vi "gfitsio-open-create-replace-image.vi"(4 "image data type":T1 items=["<invalid type>"=0, "BYTE_IMG  (U8)"=8, "SHORT_IMG  (I16)"=16, "USHORT_IMG  (U16)"=20, "LONG_IMG  (I32)"=32, "ULONG_IMG  (U32)"=40, "FLOAT_IMG  (SGL)"=-32, "DOUBLE_IMG  (DBL)"=-64], 5 "prompt (\"Select an HDU\")":string="Select an HDU", 6 "advisory dialog? (display:T)":bool=TRUE, 7 "hdu name (dialog if empty)":string, 8 "error in (no error)":errorcluster, 9 "function (open or create)":T3(ring)=enum."open or create", 10 "naxes":i32[](array[numeric]), 11 "gfits refnum":T2) -> (0 "error out":errorcluster, 2 "hdu name out":string, 3 "dup gfits refnum":T2)   [LabVIEW 2019, in "gfitsio.lvlib"]
doc: "Opens an existing FITS image HDU, creates a new FITS image HDU, or replaces an existing FITS image HDU, programmatically or interactively using a dialog box. You can optionally specify a dialog prompt."
uses:
  gfitsio.lvlib
  gfitsio-refnum.ctl
  cfitsio-bitpix.ctl
  cfitsio-hdutypes.ctl
  gfitsio-error-codes.ctl
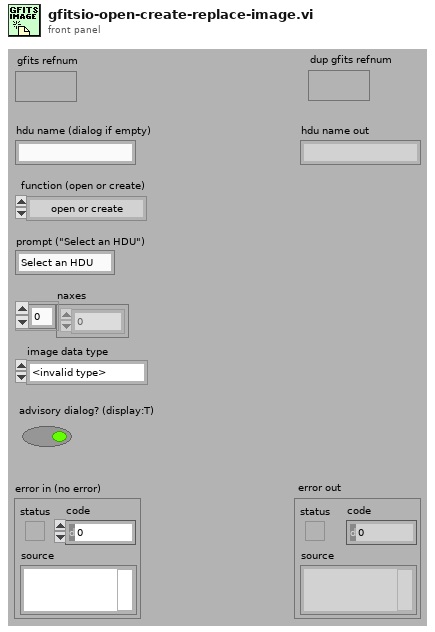
[diagram p1: front panel]
types:
  T1 = typedef "gfitsio.lvlib/cfitsio-bitpix.ctl" = i32
  T2 = typedef "gfitsio.lvlib/gfitsio-refnum.ctl" = refnum<k1>
  T3 = enum16{"open", "open or create", "create", "create or replace"}
  T4 = typedef "gfitsio.lvlib/cfitsio-hdutypes.ctl" = i32
  T5 = typedef "gfitsio.lvlib/gfitsio-error-codes.ctl" = i32
  T6 = enum16{"Error", "Ok", "Cancel", "Abort", "Retry", "Ignore", "Yes", "No", "Close", "Help", "Disabled"}
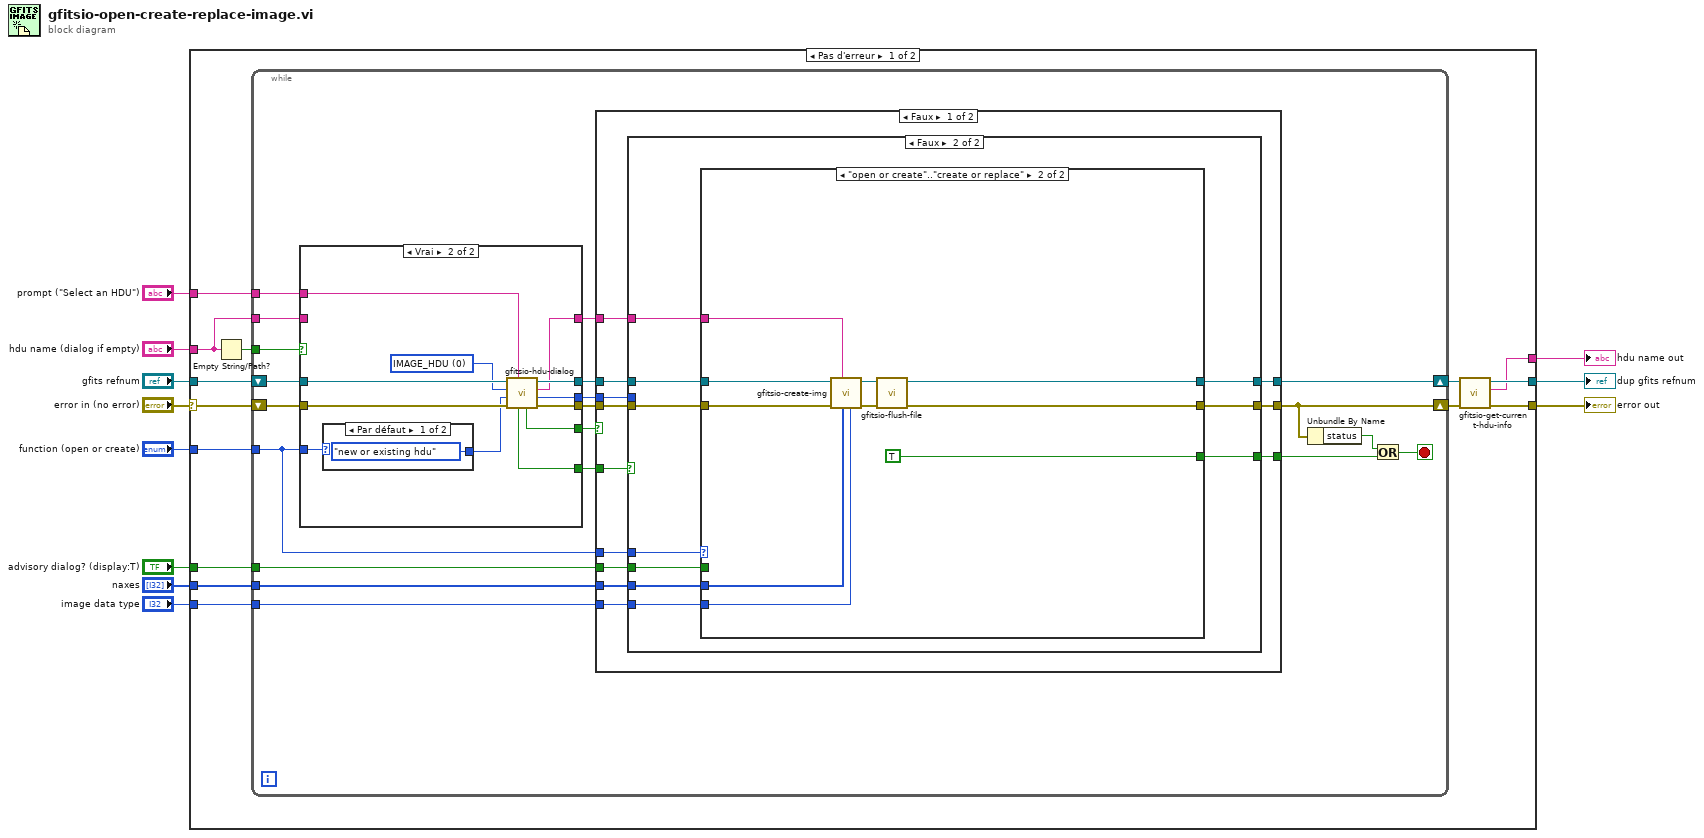
[diagram p0: block diagram]
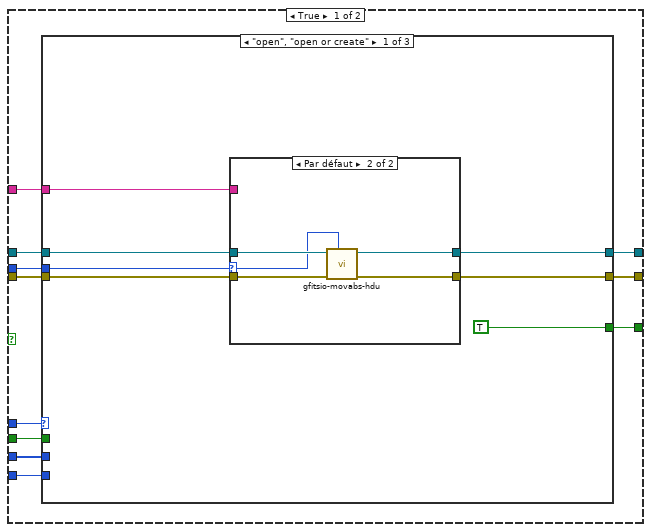
[diagram p2: hidden frame]
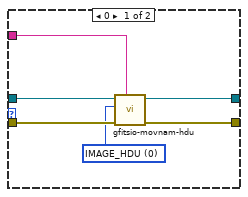
[diagram p3: hidden frame]
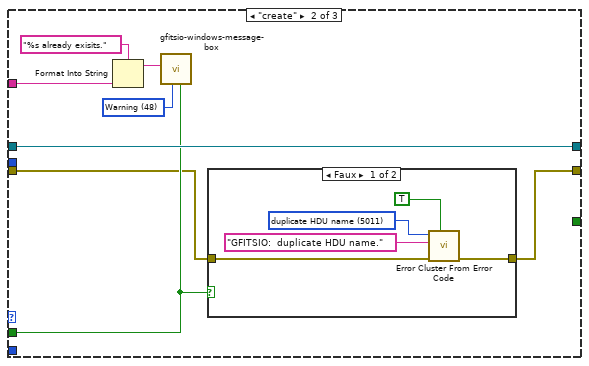
[diagram p4: hidden frame]
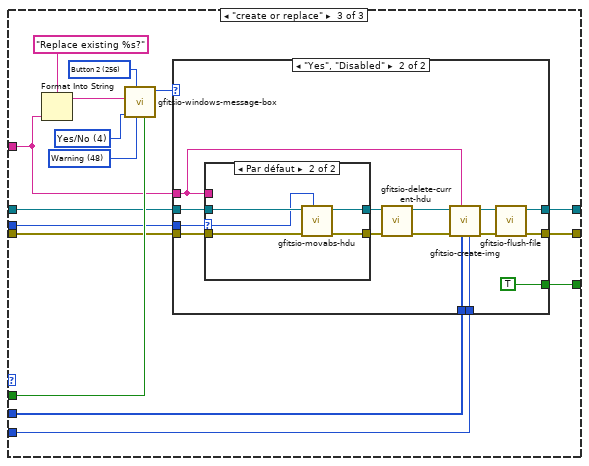
[diagram p6: hidden frame]
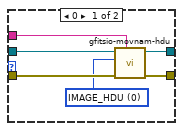
[diagram p8: hidden frame]
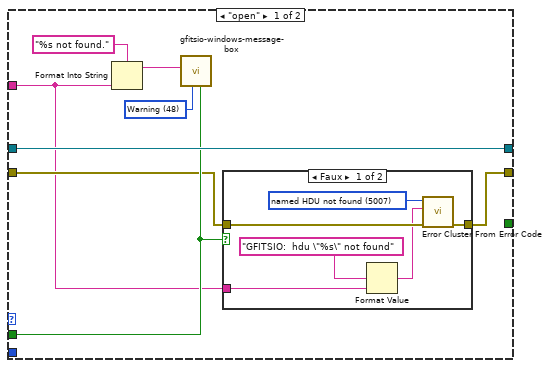
[diagram p9: hidden frame]
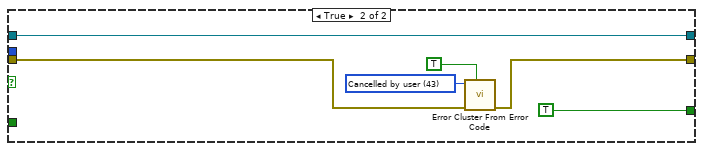
[diagram p11: hidden frame]
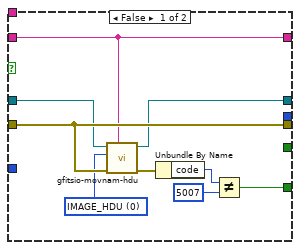
[diagram p12: hidden frame]
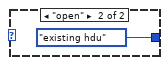
[diagram p13: hidden frame]
diagram:
  n1 = case shown="Pas d'erreur" "error in (no error)" {
    selector: "error in (no error)" -> [w12 w209]
    tunnel: "advisory dialog? (display:T)" -> [w24 _]
    tunnel: "function (open or create)" -> [w23 _]
    tunnel: "prompt (\"Select an HDU\")" -> [w22 _]
    tunnel: "hdu name (dialog if empty)" -> [w21 _]
    tunnel: "gfits refnum" -> [w20 w210]
    tunnel: [w17 w209] -> w6
    tunnel: [w16 w210] -> w5
    tunnel: [w15 _] -> w4
    tunnel: "naxes" -> [w14 _]
    tunnel: "image data type" -> [w13 _]
    frame No Error {
      n2 = Empty String/Path?(string/path=w21) -> (empty?=w25:bool)
      n3 = while {
        tunnel: w23 -> [w29]
        tunnel: w25 -> [w43]
        shift-right: [w38] -> w18
        shift-left: w12 -> [w45]
        shift-right: [w41] -> w19
        shift-left: w20 -> [w44]
        tunnel: w21 -> [w33]
        tunnel: w22 -> [w30]
        tunnel: w24 -> [w28]
        tunnel: w14 -> [w27]
        tunnel: w13 -> [w26]
        stop <- w35 stop-if-true
        n4 = case shown="Vrai" w43 {
          tunnel: [w194 w206] -> w40
          tunnel: [w192 w205] -> w42
          tunnel: w45 -> [w194 w204]
          tunnel: w44 -> [w193 w203]
          tunnel: w29 -> [_ w202]
          tunnel: [_ w201] -> w39
          tunnel: [w188 w200] -> w34
          tunnel: w33 -> [w187 _]
          tunnel: [w187 w199] -> w32
          tunnel: [_ w198] -> w31
          tunnel: w30 -> [_ w197]
          frame False {
            w186 = T4 0 items=["ANY_HDU"=-1, "IMAGE_HDU"=0, "ASCII_TBL"=1, "BINARY_TBL"=2] ("hdu type (ANY)")
            n5 = call "gfitsio-movnam-hdu.vi"("extname"=w187, "error in (no error)"=w194, "hdutype (ANY_HDU)"=w186, "gfits refnum"=w193) -> ("error out"=w191:errorcluster, "dup gfits refnum"=w192:T2)  [unwired: 6 in]
            n6 = Unbundle By Name(w191) -> ("code"=w190:i32)
            n7 = Not Equal?(x=w190, y=5007) -> (x != y?=w188:bool)
          }
          frame True {
            w195 = T4 0 items=["ANY_HDU"=-1, "IMAGE_HDU"=0, "ASCII_TBL"=1, "BINARY_TBL"=2] ("hdu type (ANY)")
            n8 = case shown="Par défaut" w202 {
              tunnel: [enum32{"existing hdu", "new or existing hdu"}."new or existing hdu" ("select mode (new or existing)") enum32{"existing hdu", "new or existing hdu"}."existing hdu" ("select mode (new or existing)")] -> w196
              frame Default {
              }
              frame "open" {
              }
            }
            n9 = call "gfitsio-hdu-dialog.vi"("prompt (\"Select an HDU\")"=w197, "error in (no error)"=w204, "select mode (new or existing)"=w196, "hdu type (ANY_HDU)"=w195, "gfits refnum"=w203) -> ("error out"=w206:errorcluster, "hdu number (0 if cancelled)"=w198:i32, "hdu name (\"\" if cancelled)"=w199:string, "dup gfits refnum"=w205:T2, "cancelled"=w201:bool, "exists"=w200:bool)  [unwired: 1 in]
          }
        }
        n10 = case shown="Faux" w39 {
          tunnel: w42 -> [w57 w185]
          tunnel: [w54 w185] -> w41
          tunnel: w40 -> [w56 w181]
          tunnel: [w55 w180] -> w38
          tunnel: [w48 TRUE] -> w36
          tunnel: w34 -> [w53 _]
          tunnel: w32 -> [w51 _]
          tunnel: w31 -> [w50 _]
          tunnel: w29 -> [w52 _]
          tunnel: w28 -> [w49 _]
          tunnel: w27 -> [w47 _]
          tunnel: w26 -> [w46 _]
          frame False {
            n11 = case shown="Faux" w53 {
              tunnel: w57 -> [w67 w153]
              tunnel: w56 -> [w64 w152]
              tunnel: [w65 w151] -> w55
              tunnel: [w66 w150] -> w54
              tunnel: w52 -> [w68 w154]
              tunnel: w51 -> [w63 w148]
              tunnel: w50 -> [w62 _]
              tunnel: w49 -> [w61 w149]
              tunnel: [w60 w147] -> w48
              tunnel: w47 -> [w59 w146]
              tunnel: w46 -> [w58 w145]
              frame True {
                n12 = case shown="\"open\", \"open or create\"" w68 {
                  tunnel: w67 -> [w74 w94 w110]
                  tunnel: [w72 w94 w109] -> w66
                  tunnel: [w73 w87 w107] -> w65
                  tunnel: w64 -> [w75 w88 w108]
                  tunnel: w63 -> [w71 w90 w104]
                  tunnel: w62 -> [w70 _ w103]
                  tunnel: w61 -> [_ w89 w111]
                  tunnel: [TRUE _ w105] -> w60
                  tunnel: w59 -> [_ _ w102]
                  tunnel: w58 -> [_ _ w101]
                  frame "open", "open or create" {
                    n13 = case shown="Par défaut" w70 {
                      selector: w70 -> [_ w82]
                      tunnel: w75 -> [w81 w85]
                      tunnel: w74 -> [w80 w86]
                      tunnel: [w79 w84] -> w73
                      tunnel: [w78 w83] -> w72
                      tunnel: w71 -> [w77 _]
                      frame 0 {
                        w76 = T4 0 items=["ANY_HDU"=-1, "IMAGE_HDU"=0, "ASCII_TBL"=1, "BINARY_TBL"=2] ("hdu type (ANY)")
                        n14 = call "gfitsio-movnam-hdu.vi"("extname"=w77, "error in (no error)"=w81, "hdutype (ANY_HDU)"=w76, "gfits refnum"=w80) -> ("error out"=w79:errorcluster, "dup gfits refnum"=w78:T2)  [unwired: 6 in]
                      }
                      frame Default {
                        n15 = call "gfitsio-movabs-hdu.vi"("hdunum"=w82, "error in (no error)"=w85, "gfits refnum"=w86) -> ("error out"=w84:errorcluster, "dup gfits refnum"=w83:T2)  [unwired: 6 in, 1 out]
                      }
                    }
                  }
                  frame "create" {
                    w91 = u32 48 items=["None"=0, "Warning"=48, "Confirmation"=64, "Question"=32, "Error"=16, "User Icon"=128] ("Icon (None)")
                    n16 = Format Into String(format string="%s already exisits.", w90) -> (resulting string=w92:string)  [unwired: 2 in, 1 out]
                    n17 = call "gfitsio-windows-message-box.vi"("enable dialog?"=w89, "Icon (None)"=w91, "Text"=w92) -> ()  [unwired: 8 in, 1 out]
                    n18 = case shown="Faux" w89 {
                      tunnel: w88 -> [w99 w100]
                      tunnel: [w98 w100] -> w87
                      frame False {
                        w95 = T5 5011 items=["no error"=0, "dimensionality conflict"=5001, "fpixel out of image bounds"=5002, "lpixel out of image bounds"=5003, "increment size larger than image"=5004, "increment must be greater than zero"=5005, "fpixel must specify lower left corner"=5006, "named HDU not found"=5007, "specified row is past the end of the table"=5008, "wrong number of elements for column"=5009, "column is not scalar"=5010, "duplicate HDU name"=5011, "invalid table type"=5012] ("Ring")
                        n19 = call <vilib>:"Error Cluster From Error Code.vi"("show call chain? (False)"=TRUE, "error in (no error)"=w99, "error message (\"\")"="GFITSIO:  duplicate HDU name." ("error message (\"\")"), "error code (0)"=w95) -> ("error out"=w98:errorcluster)  [unwired: 5 in]
                      }
                      frame True {
                      }
                    }
                  }
                  frame "create or replace" {
                    w113 = u32 256 items=["Button 1"=0, "Button 2"=256, "Button 3"=512, "Button 4"=1024] ("Default (Button 1)")
                    w114 = u32 4 items=["Abort/Retry/Ignore"=2, "OK"=0, "OK/Cancel"=1, "Retry/Cancel"=5, "Yes/No"=4, "Yes/No/Cancel"=3] ("Buttons (OK)")
                    w115 = u32 48 items=["None"=0, "Warning"=48, "Confirmation"=64, "Question"=32, "Error"=16, "User Icon"=128] ("Icon (None)")
                    n20 = Format Into String(format string="Replace existing %s?", w104) -> (resulting string=w112:string)  [unwired: 2 in, 1 out]
                    n21 = call "gfitsio-windows-message-box.vi"("enable dialog?"=w111, "Icon (None)"=w115, "Default (Button 1)"=w113, "Buttons (OK)"=w114, "Text"=w112) -> ("Button Selected"=w106:T6)  [unwired: 6 in]
                    n22 = case shown="\"Yes\", \"Disabled\"" w106 {
                      tunnel: w110 -> [w118 w132]
                      tunnel: [w118 w123] -> w109
                      tunnel: w108 -> [w117 w131]
                      tunnel: [w117 w122] -> w107
                      tunnel: [_ TRUE] -> w105
                      tunnel: w104 -> [_ w121]
                      tunnel: w103 -> [_ w130]
                      tunnel: w102 -> [_ w120]
                      tunnel: w101 -> [_ w119]
                      frame "No", Default {
                      }
                      frame "Yes", "Disabled" {
                        n23 = case shown="Par défaut" w130 {
                          selector: w130 -> [_ w140]
                          tunnel: w131 -> [w139 w143]
                          tunnel: w132 -> [w138 w144]
                          tunnel: [w137 w142] -> w129
                          tunnel: [w136 w141] -> w128
                          tunnel: w121 -> [w135 _]
                          frame 0 {
                            w134 = T4 0 items=["ANY_HDU"=-1, "IMAGE_HDU"=0, "ASCII_TBL"=1, "BINARY_TBL"=2] ("hdu type (ANY)")
                            n24 = call "gfitsio-movnam-hdu.vi"("extname"=w135, "error in (no error)"=w139, "hdutype (ANY_HDU)"=w134, "gfits refnum"=w138) -> ("error out"=w137:errorcluster, "dup gfits refnum"=w136:T2)  [unwired: 6 in]
                          }
                          frame Default {
                            n25 = call "gfitsio-movabs-hdu.vi"("hdunum"=w140, "error in (no error)"=w143, "gfits refnum"=w144) -> ("error out"=w142:errorcluster, "dup gfits refnum"=w141:T2)  [unwired: 6 in, 1 out]
                          }
                        }
                        n26 = call "gfitsio-delete-current-hdu.vi"("error in (no error)"=w129, "gfits refnum"=w128) -> ("error out"=w126:errorcluster, "dup gfits refnum"=w127:T2)  [unwired: 8 in]
                        n27 = call "gfitsio-create-img.vi"("image data type"=w119, "naxes"=w120, "extname"=w121, "error in (no error)"=w126, "gfits refnum"=w127) -> ("error out"=w125:errorcluster, "dup gfits refnum"=w124:T2)  [unwired: 5 in]
                        n28 = call "gfitsio-flush-file.vi"("error in (no error)"=w125, "gfits refnum"=w124) -> ("error out"=w122:errorcluster, "dup gfits refnum"=w123:T2)  [unwired: 8 in]
                      }
                    }
                  }
                }
              }
              frame False {
                n29 = case shown="\"open or create\"..\"create or replace\"" w154 {
                  tunnel: w153 -> [w162 w178]
                  tunnel: w152 -> [w157 w179]
                  tunnel: [w156 w174] -> w151
                  tunnel: [w162 w173] -> w150
                  tunnel: w149 -> [w158 _]
                  tunnel: w148 -> [w155 w172]
                  tunnel: [_ TRUE] -> w147
                  tunnel: w146 -> [_ w171]
                  tunnel: w145 -> [_ w170]
                  frame "open" {
                    w159 = u32 48 items=["None"=0, "Warning"=48, "Confirmation"=64, "Question"=32, "Error"=16, "User Icon"=128] ("Icon (None)")
                    n30 = Format Into String(format string="%s not found.", w155) -> (resulting string=w160:string)  [unwired: 2 in, 1 out]
                    n31 = call "gfitsio-windows-message-box.vi"("enable dialog?"=w158, "Icon (None)"=w159, "Text"=w160) -> ()  [unwired: 8 in, 1 out]
                    n32 = case shown="Faux" w158 {
                      tunnel: w157 -> [w168 w169]
                      tunnel: [w167 w169] -> w156
                      tunnel: w155 -> [w165 _]
                      frame False {
                        w163 = T5 5007 items=["no error"=0, "dimensionality conflict"=5001, "fpixel out of image bounds"=5002, "lpixel out of image bounds"=5003, "increment size larger than image"=5004, "increment must be greater than zero"=5005, "fpixel must specify lower left corner"=5006, "named HDU not found"=5007, "specified row is past the end of the table"=5008, "wrong number of elements for column"=5009, "column is not scalar"=5010, "duplicate HDU name"=5011, "invalid table type"=5012] ("Ring")
                        n33 = Format Value(format string="GFITSIO:  hdu \"%s\" not found", value (0)=w165) -> (output string=w164:string)  [unwired: 1 in]
                        n34 = call <vilib>:"Error Cluster From Error Code.vi"("error in (no error)"=w168, "error message (\"\")"=w164, "error code (0)"=w163) -> ("error out"=w167:errorcluster)  [unwired: 6 in]
                      }
                      frame True {
                      }
                    }
                  }
                  frame "open or create".."create or replace" {
                    n35 = call "gfitsio-create-img.vi"("image data type"=w170, "naxes"=w171, "extname"=w172, "error in (no error)"=w179, "gfits refnum"=w178) -> ("error out"=w176:errorcluster, "dup gfits refnum"=w175:T2)  [unwired: 5 in]
                    n36 = call "gfitsio-flush-file.vi"("error in (no error)"=w176, "gfits refnum"=w175) -> ("error out"=w174:errorcluster, "dup gfits refnum"=w173:T2)  [unwired: 8 in]
                  }
                }
              }
            }
          }
          frame True {
            w183 = 43 items=["No error", "Argument error", "Memory is full", "Out of zone", "End of file", "File already open", "Generic file I/O error", "File not found", "File permission error", "Disk is full", "Duplicate path", "Too many files open", "System feature not enabled", "Resource file not found", "Cannot add resource", "Resource not found", "Image not found", "Image memory error", "Pen does not exist", "Config type invalid", "Config token not found", "Config parse error", "Config memory error", "Bad external code format", "Bad external code offset", "External code not present", "Null window", "Destroy window error", "Null menu", "Print aborted", "Bad print record", "Print driver error", "Windows error during printing", "Memory error during printing", "Print dialog error", "Generic print error", "Invalid device refnum", "Device not found", "Device parameter error", "Device unit error", "Cannot open device", "Device call aborted", "Generic error", "Cancelled by user", "Object ID too low", "Object ID too high", "Object not in heap", "Unknown heap", "Unknown object (invalid DefProc)", "Unknown object (DefProc not in table)", "Message out of range", "Invalid (null) method", "Unknown message", "Manager call not supported", "Bad address", "Network operation in progress", "Network operation timed out", "Connection is busy", "Network attribute not supported", "Network error", "Address in use", "System out of memory", "Connection aborted", "Connection refused", "Not connected", "Already connected", "Connection closed", "Initialization error (interapplication manager)", "Bad occurrence", "Wait on unbound occurrence handler", "Occurrence queue overflow", "Datalog type conflict", "Unused", "Unrecognized type (interapplication manager)", "Memory corrupt", "Failed to make temporary DLL", "Old CIN version", "Drag socket not found", "Failed to load drop-object", "Failed to register OLE object", "Failed to release OLE object", "Format specifier type mismatch", "Unknown format specifier", "Too few format specifiers", "Too many format specifiers", "Scan failed", "Newer CIN version", "Error converting to variant", "Runtime menu error", "Password tampered", "Variant attribute not found", "Incompatible variant data type", "Event data is not available", "Event Store is not present", "Occurrence is not found", "Event Queue is not created", "Event info is not available in the type library", "Refnum passed is NULL", "Error retrieving Class GUID", "Error retrieving CoClass GUID", "Error retrieving TypeLib GUID.", "Bad built application magic bytes.", "Specific driver is different from the specific driver associated with the Logical Name.", "There is no session opened to the class driver.", "Max Error", "MAX - Error with config objects", "MAX - Error loading configuration", "MAX - Group not supported", "Singlecast connections can not send to multicast addresses.", "Multicast connections can not send to singlecast addresses.", "Specified IP address not in multicast address range.", "Attempt to write to read-only multicast connection.", "Attempt to read from write-only multicast connection.", "The buffer used to receive a datagram was smaller than the datagram itself"]
            n37 = call <vilib>:"Error Cluster From Error Code.vi"("show call chain? (False)"=TRUE, "error in (no error)"=w181, "error code (0)"=w183) -> ("error out"=w180:errorcluster)  [unwired: 6 in]
          }
        }
        n38 = Unbundle By Name(w38) -> ("status"=w37:bool)
        n39 = Or(x=w37, y=w36) -> (x .or. y?=w35:bool)
      }
      n40 = call "gfitsio-get-current-hdu-info.vi"("error in (no error)"=w18, "gfits refnum"=w19) -> ("error out"=w17:errorcluster, "hdu name"=w15:string, "dup gfits refnum"=w16:T2)  [unwired: 5 in, 2 out]
    }
    frame Error {
    }
  }
  "error out" <- w6
  "dup gfits refnum" <- w5
  "hdu name out" <- w4
